vi "CH_LM Communication Dialog.vi"() -> (0 "OK":bool, 1 "Communication Mode":T1, 2 "GPIB Board":i16)   [LabVIEW 2012, in "CH_LM App.lvlib"]
doc: "This dialog VI asks the user for communication mode and additional paramters."
uses:
  CH_LM App.lvlib
  CH_LM/CH_LM Communication Mode.ctl
  CH_LM.lvlib
panel:
  in  "stop":bool
  in  "OK Button":bool
  in  "GPIB Board (0)":i16
  in  "Communication Mode":T1
  # "Please, specify communication mode and\nGPIB board ID in case of GPIB or\nSerial Configuration in case of RS232."
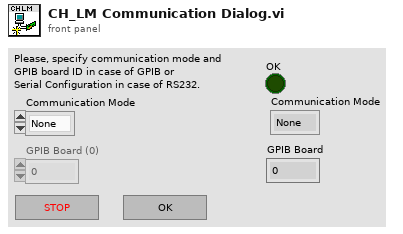
[diagram p1: front panel]
types:
  T1 = typedef "CH_LM.lvlib/CH_LM Communication Mode.ctl" = enum16{"None", "USB", "GPIB", "RS232"}
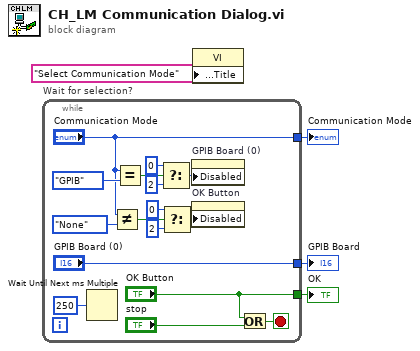
[diagram p0: block diagram]
diagram:
  n1 = while "Wait for selection?" {
    tunnel: ["OK Button"] -> w2
    tunnel: ["GPIB Board (0)"] -> w3
    tunnel: ["Communication Mode"] -> w4
    stop <- w20 stop-if-true
    n2 = Wait Until Next ms Multiple(millisecond multiple=u32 250) -> ()  [unwired: 1 out]
    n3 = Not Equal?(x="Communication Mode", y=CH_LM_Communication_Mode."None") -> (x != y?=w6:bool)
    n4 = Equal?(x="Communication Mode", y=CH_LM_Communication_Mode."GPIB" ("Communication Mode")) -> (x = y?=w14:bool)
    n5 = Select(t=u8 0 ("Disabled"), s=w14, f=u8 2 ("Disabled")) -> (s? t:f=w13:u8)
    n6 = Select(t=u8 0 ("Disabled"), s=w6, f=u8 2 ("Disabled")) -> (s? t:f=w8:u8)
    n7 = property on="GPIB Board (0)" class="DigNum (strict)"("Disabled"=w13) -> ()  [unwired: 2 in, 2 out]
    n8 = property on="OK Button" class="Bool"("Disabled"=w8) -> ()  [unwired: 2 in, 2 out]
    n9 = Or(x="OK Button", y="stop") -> (x .or. y?=w20:bool)
  }
  "Communication Mode" <- w4
  "GPIB Board" <- w3
  "OK" <- w2
  n10 = property class="VI"("Front Panel Window:Title"="Select Communication Mode") -> ()  [unwired: 2 in, 2 out]
